vi "Dashboard Main.vi"() -> ()   [LabVIEW 2015]
uses:
  Vision/Vision Support Code/Camera Types.ctl
  <vilib>/Rock Robotics/WPI/Camera/WPI_CameraImageSize.ctl
  <vilib>/Utility/miscctls.llb/LVRowAndColumnTypeDef.ctl
  <vilib>/event_ctls.llb/eventvkey.ctl
  <vilib>/Rock Robotics/WPI/Dashboard/WPI_DashboardLogging Global.vi
  Vision/Robot Global Data.vi
  <vilib>/Rock Robotics/Network Tables/NT Read Numeric Array.vi
  <vilib>/Rock Robotics/Network Tables/NT Read Boolean.vi
  <vilib>/Rock Robotics/Network Tables/NT Write Boolean.vi
  <vilib>/Utility/config.llb/Write Key (String).vi
  <vilib>/Utility/config.llb/Write Key (I32).vi
  <vilib>/Utility/config.llb/NI_LVConfig.lvlib
  <vilib>/vision/NI_Vision_Development_Module.lvlib
panel:
  in  "Tab Control":T1(tab)
  out "Boolean 4":bool
  out "Boolean 3":bool
  out "Boolean 2":bool
  out "Boolean":bool
  out "Original Image":T2(plugin-control)
  out "Masked":T2(plugin-control)
  out "Detected Targets":T3(array[cluster]) {"Normalized Rect"."Numeric 5" format="%#_2g"; "Normalized Rect"."Numeric 3" format="%#_2g"; "Normalized Rect"."Numeric 2" format="%#_2g"; "Normalized Rect"."Numeric" format="%#_2g"}
  out "Sorted Particle Scores":T4(array[cluster]) {"Moment Factor" format="%#_3g"; "Aspect Ratio" format="%#_3g"; "Area to CH" format="%#_3g"; "X" format="%#_3g"; "Y" format="%#_3g"}
  in  "LED Color":T5={"Hue"={98.0, 128.0}, "Sat"={64.0, 255.0}, "Val"={48.571428571428584, 255.0}} {"Hue" scale=0.0..255.0 scale format="%#_3g"}
  in  "Display Original":bool=TRUE
  in  "Display Mask":bool=TRUE
  in  "Emphasize Limit Tests":bool=TRUE
  in  "Camera Type":T6=enum."MS HD3000 square"
  in  "Aspect Fudge Factor":dbl=1.0
  in  "Score Threshold":dbl=75.0
  in  "Image Size":T7=enum."320x240"
  out "Qualified Particles":i32
  out "Highest Avg Score":dbl
  in  "Min Score Threshold":i32=75
  out "NT Connection":bool
  out "fps":dbl format="%#.1g"
  out "Mbps":dbl format="%#.1g"
  out "Mbps LED":bool
  in  "TCP":refnum<k5>
  in  "Rec Mode":enum32{"Stop", "Record", "Playback"}(radio)
  in  "Vision":u16(ring)=2 items=["Camera Off", "USB Camera SW", "USB Camera HW", "IP Camera"]
  out "Camera IP":string
  out "Image Message":string="Timeout in Camera Communications"
  in  "Dashboard Tab":T8(tab)
  out "Ball Holder OR":bool
  out "Shooter":bool
  out "Intake":bool
  in  "Gyro Reset":bool
  out "Gyro":dbl
  in  "OW Arm Angle":dbl=42.0
  out "Wheels Good":bool
  out "Arm Good":bool
  in  "Auto Selection":u16(ring) caption="Menu Ring" items=["Do Nothing", "Bump", "CDF", "Low Bar", "Bump - SHOOT", "Bump - SHOOT DRIVE", "CDF - SHOOT", "Low Bar - SHOOT", "Spy - SHOOT", "Misc Auto 1"]
  out "VISION GOOD":bool
  out "Arm Angle":dbl
  out "Encoder Distance":dbl
  out "RPM L":dbl
  out "RPM R":dbl
  out "RPM SP":dbl
  out "Angle SP":dbl
  out "Found Targets":cluster{dbl, dbl}
  in  "Vision Good Range":dbl=0.05
  in  "Vision Scaling":dbl
  in  "148 Arm Angle":dbl=60.0
  out "Encoder Gyro":dbl
  out "Gyro":dbl(knob) scale=0.0..360.0
  in  "D4 Wheel Speed":dbl=5000.0
  in  "Fender Wheel Speed":dbl=4999.0
  in  "Select Auto":string(combo)
  in  "Camera Settings":T9={"Frame Rate"=30, "Compression"=30, "Size"=1} {"Frame Rate" scale=1.0..30.0; "Size" items=["640x480", "320x240", "160x120"]}
  out "MotorChart R":cluster{"Numeric":dbl, "Numeric":dbl}(graph)
  out "MotorChart L":T10(graph)
  out "MotorSliders R":cluster{"MotorSlide1":dbl, "MotorSlide2":dbl} {"MotorSlide2" scale=-1.0..1.0 scale format="%#_2e"; "MotorSlide1" scale=-1.0..1.0 scale format="%#_2e"}
  out "MotorSliders L":T11 {"MotorSlide4 2" scale=0.0..14.0 scale format="%#_2e"; "MotorSlide2" scale=-1.0..1.0 scale format="%#_2e"; "MotorSlide1" scale=-1.0..1.0 scale format="%#_2e"}
  out "JS1 Z":dbl(slide) scale=-1.0..1.0 scale format="%#_2e"
  out "JS1 Graph":cluster{"X":dbl, "Y":dbl}[](graph)
  out "JS1 Buttons":T12
  out "JS2 Z":dbl(slide) scale=-1.0..1.0 scale format="%#_2e"
  out "JS2 Graph":cluster{"X":dbl, "Y":dbl}[](graph)
  out "JS2 Buttons":T12
  out "Mode":T13(ring)=enum."Auto Disabled"
  in  "DB Camera Config":bool
  in  "DB/String 9":string
  in  "DB/String 8":string
  in  "DB/String 7":string
  in  "DB/String 6":string
  in  "DB/String 5":string
  in  "DB/String 4":string
  in  "DB/String 3":string
  in  "DB/String 2":string
  in  "DB/String 1":string
  in  "DB/String 0":string
  in  "DB/Slider 0":dbl(slide) scale=0.0..5.0
  in  "DB/Slider 1":dbl(slide) scale=0.0..5.0
  in  "DB/Slider 2":dbl(slide) scale=0.0..5.0
  in  "DB/Slider 3":dbl(slide) scale=0.0..5.0
  out "DB/LED 3":bool
  out "DB/LED 2":bool
  out "DB/LED 1":bool
  out "DB/LED 0":bool
  in  "DB/Button 3":bool
  in  "DB/Button 2":bool
  in  "DB/Button 1":bool
  in  "DB/Button 0":bool caption="New Name"
  in  "Test Slider":dbl(slide) scale=0.0..100.0 scale format="%#_3g"
  in  "On/Off":bool caption="Solenoid"
  in  "Test Name":u16(ring) items=["Select the test to run..."]
  in  "Test Tree":string(tree)
  in  "Motor":cluster{"Value":dbl, "Enable":bool} {"Value" scale=-1.0..1.0 scale format="%#_3g"}
  out "Progress":T14 {"Test Progress" scale=0.0..100.0}
  in  "Rev/Fwd":cluster{"Forward":bool, "Reverse":bool}
  in  "Test Ring":u16(ring) items=["Monochrome", "Color"]
  out "Cmd Status":string
  in  "Execute Command":bool
  in  "Command Params":string[][](table)
  in  "Command Selection":i32(listbox)
  in  "CheckList":i32(listbox)
  out "Tree":string(tree)
  # "Density Profile"
  # "Left"
  # "Front"
  # "Right"
  # "Battery"
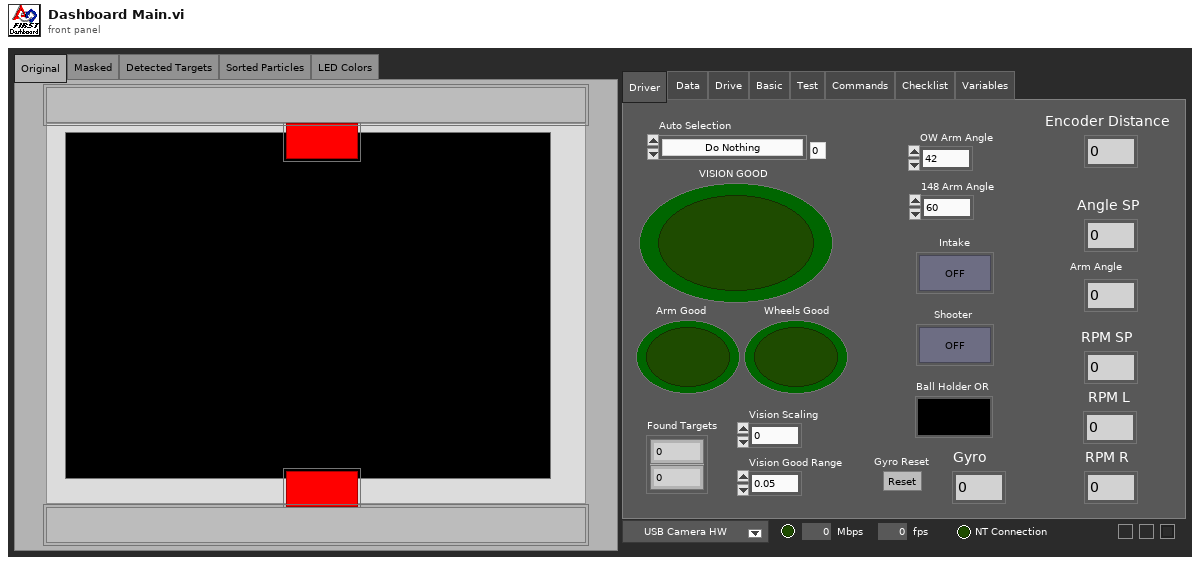
[diagram p1: front panel]
types:
  T1 = enum32{"Original", "Masked", "Detected Targets", "Sorted Particles", "LED Colors"}
  T2 = typedef "IMAQ Image.ctl" = refnum<image>
  T3 = cluster{"Distance (ft)":dbl, "Center":cluster{dbl, dbl}, "Normalized Rect":cluster{"Numeric":dbl, "Numeric 2":dbl, "Numeric 3":dbl, "Numeric 5":dbl}}[]
  T4 = cluster{"Rectangle px":cluster{"Numeric":dbl, "Numeric 2":dbl, "Numeric 3":dbl, "Numeric 5":dbl}, "Aspect Ratio":dbl, "Area to CH":dbl, "X":dbl, "Y":dbl, "Moment Factor":dbl}[]
  T5 = cluster{"Hue":cluster{dbl, dbl}, "Sat":cluster{dbl, dbl}, "Val":cluster{dbl, dbl}}
  T6 = typedef "Camera Types.ctl" = enum16{"206", "1011", "1013", "MS HD3000 square", "MS HD3000 640x480"}
  T7 = typedef "WPI_CameraImageSize.ctl" = enum16{"640x480", "320x240", "160x120", "Custom"}
  T8 = enum32{"Driver", "Data ", "Drive", "Basic", "Test", "Commands", "Checklist", "Variables"}
  T9 = cluster{"Frame Rate":i32, "Compression":i32, "Size":u16}
  T10 = cluster{"Numeric":dbl, "Numeric":dbl, "Battery V":dbl}
  T11 = cluster{"MotorSlide1":dbl, "MotorSlide2":dbl, "MotorSlide4 2":dbl}
  T12 = cluster{bool, bool, bool, bool, bool, bool, bool, bool, bool, bool, bool, bool}
  T13 = enum8{"Tele-Op Disabled", "Tele-Op Enabled", "Auto Disabled", "Auto Enabled", "Test Disabled", "Test Enabled", "Disconnected", "No Code", "E-Stop"}
  T14 = cluster{"Test Progress":u8, "Test Progress Text":string}
  T15 = typedef "Image Type" = u32
  T16 = typedef "Particle Parameters" = i32
  T17 = cluster{"IDs":cluster{"RPC field ID":u16, "Unique ID":u16}, "String":string}
  T18 = enum32{"Drive", "Basic", "Custom", "Test", "Checklist", "Variables"}
  T19 = cluster{"Bounding box":cluster{"left":dbl, "top":dbl, "right":dbl, "bottom":dbl}, "Aspect Ratio":dbl, "Area to CH":dbl, "X Mask":dbl, "Y Mask":dbl, "Moment":dbl}[]
  T20 = cluster{"Rectangle":cluster{"Numeric":dbl, "Numeric 2":dbl, "Numeric 3":dbl, "Numeric 5":dbl}, "L":dbl, "Area to CH":dbl, "X":dbl, "Y":dbl, "Moment Factor":dbl}[]
  T21 = cluster{"Found Targets[0]":cluster{"Distance (ft)":dbl, "Center":cluster{dbl, dbl}, "Normalized Rect":cluster{"Numeric":dbl, "Numeric 2":dbl, "Numeric 3":dbl, "Numeric 5":dbl}}, "Found Targets[1]":cluster{"Distance (ft)":dbl, "Center":cluster{dbl, dbl}, "Normalized Rect":cluster{"Numeric":dbl, "Numeric 2":dbl, "Numeric 3":dbl, "Numeric 5":dbl}}, "Found Targets[2]":cluster{"Distance (ft)":dbl, "Center":cluster{dbl, dbl}, "Normalized Rect":cluster{"Numeric":dbl, "Numeric 2":dbl, "Numeric 3":dbl, "Numeric 5":dbl}}, "Found Targets[3]":cluster{"Distance (ft)":dbl, "Center":cluster{dbl, dbl}, "Normalized Rect":cluster{"Numeric":dbl, "Numeric 2":dbl, "Numeric 3":dbl, "Numeric 5":dbl}}, "Found Targets[4]":cluster{"Distance (ft)":dbl, "Center":cluster{dbl, dbl}, "Normalized Rect":cluster{"Numeric":dbl, "Numeric 2":dbl, "Numeric 3":dbl, "Numeric 5":dbl}}, "Found Targets[5]":cluster{"Distance (ft)":dbl, "Center":cluster{dbl, dbl}, "Normalized Rect":cluster{"Numeric":dbl, "Numeric 2":dbl, "Numeric 3":dbl, "Numeric 5":dbl}}, "Found Targets[6]":cluster{"Distance (ft)":dbl, "Center":cluster{dbl, dbl}, "Normalized Rect":cluster{"Numeric":dbl, "Numeric 2":dbl, "Numeric 3":dbl, "Numeric 5":dbl}}, "Found Targets[7]":cluster{"Distance (ft)":dbl, "Center":cluster{dbl, dbl}, "Normalized Rect":cluster{"Numeric":dbl, "Numeric 2":dbl, "Numeric 3":dbl, "Numeric 5":dbl}}, "Found Targets[8]":cluster{"Distance (ft)":dbl, "Center":cluster{dbl, dbl}, "Normalized Rect":cluster{"Numeric":dbl, "Numeric 2":dbl, "Numeric 3":dbl, "Numeric 5":dbl}}}
  T22 = typedef "NI_LVConfig.lvlib/Config Data RefNum.ctl" = refnum<k1>
  T23 = cluster{"Error Strings":string, "Disable Counts":cluster{u16, u16}, "Rail Faults":cluster{u16, u16, u16}, "Robot IP":string, "DB Mode":u8, "Event Info":cluster{"Name":string, "Type":u8, "Number":u16, "Replay":u8}, "Camera Addr":string}
  T24 = cluster{"Storage":cluster{"Disk Free":u64, "RAM Block":u32, "RAM free":u32}, "CPU Utilization":cluster{"CPU % ISR":sgl, "CPU % Time Crit":sgl, "CPU % Timed Str":sgl, "CPU % High":sgl, "CPU % Above":sgl, "CPU % Normal":sgl, "CPU % Low":sgl}, "CAN":cluster{"% Bus Utilization":sgl, "Bus Off Cnt":u32, "TX_FIFO Full Cnt":u32, "Receive Error Cnt":u8, "Transmit Error Cnt":u8}, "HID":cluster{"HID Outputs":u32, "Rumble Low":u16, "Rumble High":u16}[]}
  T25 = cluster{"Status bits":cluster{"Test Mode":bool, "Autonomous":bool, "Enabled":bool, "Code Start":bool, "Brownout":bool, "Reserved 2":bool, "Reserved 3":bool, "E-Stop":bool}, "Code Trace":cluster{"Disabled":bool, "TeleOp":bool, "Auto":bool, "Test":bool}, "Controller Type":enum16{"unknown", "cRIO", "roboRio"}, "Code?":enum16{"unknown", "noCode", "code"}, "Battery V":dbl}
  T26 = cluster{"Control Bits":cluster{"TestMode":bool, "Autonomous":bool, "Enabled":bool, "FMS Present":bool, bool, bool, bool, "E-Stop":bool}, "Team Station ":u8, "Countdown":sgl, "Joystick Values":cluster{"Axes":dbl[], "Buttons":bool[], "POVs":i16[]}[]}
  T27 = cluster{"Axes":dbl[], "Buttons":bool[], "POVs":i16[]}[]
  T28 = cluster{"Axes":dbl[], "Buttons":bool[], "POVs":i16[]}
  T29 = cluster{"Buttons[0]":bool, "Buttons[1]":bool, "Buttons[2]":bool, "Buttons[3]":bool, "Buttons[4]":bool, "Buttons[5]":bool, "Buttons[6]":bool, "Buttons[7]":bool, "Buttons[8]":bool, "Buttons[9]":bool, "Buttons[10]":bool, "Buttons[11]":bool}
  T30 = cluster{"Operation":enum16{"Update", "Clear"}, "Color Box":u32}[]
  T31 = typedef "eventvkey.ctl" = enum16{"ASCII", "Enter", "Return", "Shift", "Ctrl", "Alt", "Cmd", "Opt", "Caps", "NumLock", "Clear", "Break", "Up", "Down", "Left", "Right", "Insert", "Delete", "Home", "End", "PageUp", "PageDown", "Escape", "Help", "Pause", "ScrollLock", "F1", "F2", "F3", "F4", "F5", "F6", "F7", "F8", "F9", "F10", "F11", "F12", "F13", "F14", "F15", "F16", "F17", "F18", "F19", "F20", "F21", "F22", "F23", "F24", "Play", "VolumeUp", "VolumeDown", "Mute", "Two Byte Char"}
  T32 = cluster{"Image Size":bool, "Image Type":bool, "Pixel Value":bool, "ROI Information":bool, "Zoom Factor":bool}
  T33 = enum8{"Enabled", "Disabled", "Disabled and Grayed Out"}
  T34 = cluster{"Operation":enum16{"Update", "Clear"}, "Color Box":u32}
  T35 = typedef "LVRowAndColumnTypeDef.ctl" = cluster{"Row":i32, "Column":i32}
  T36 = cluster{"Shift":bool, "Ctrl":bool, "Alt":bool, "Cmd":bool, "Opt":bool}
  T37 = enum32{"Drive", "Basic", "Custom", "Test", "Commands", "Checklist", "Variables"}
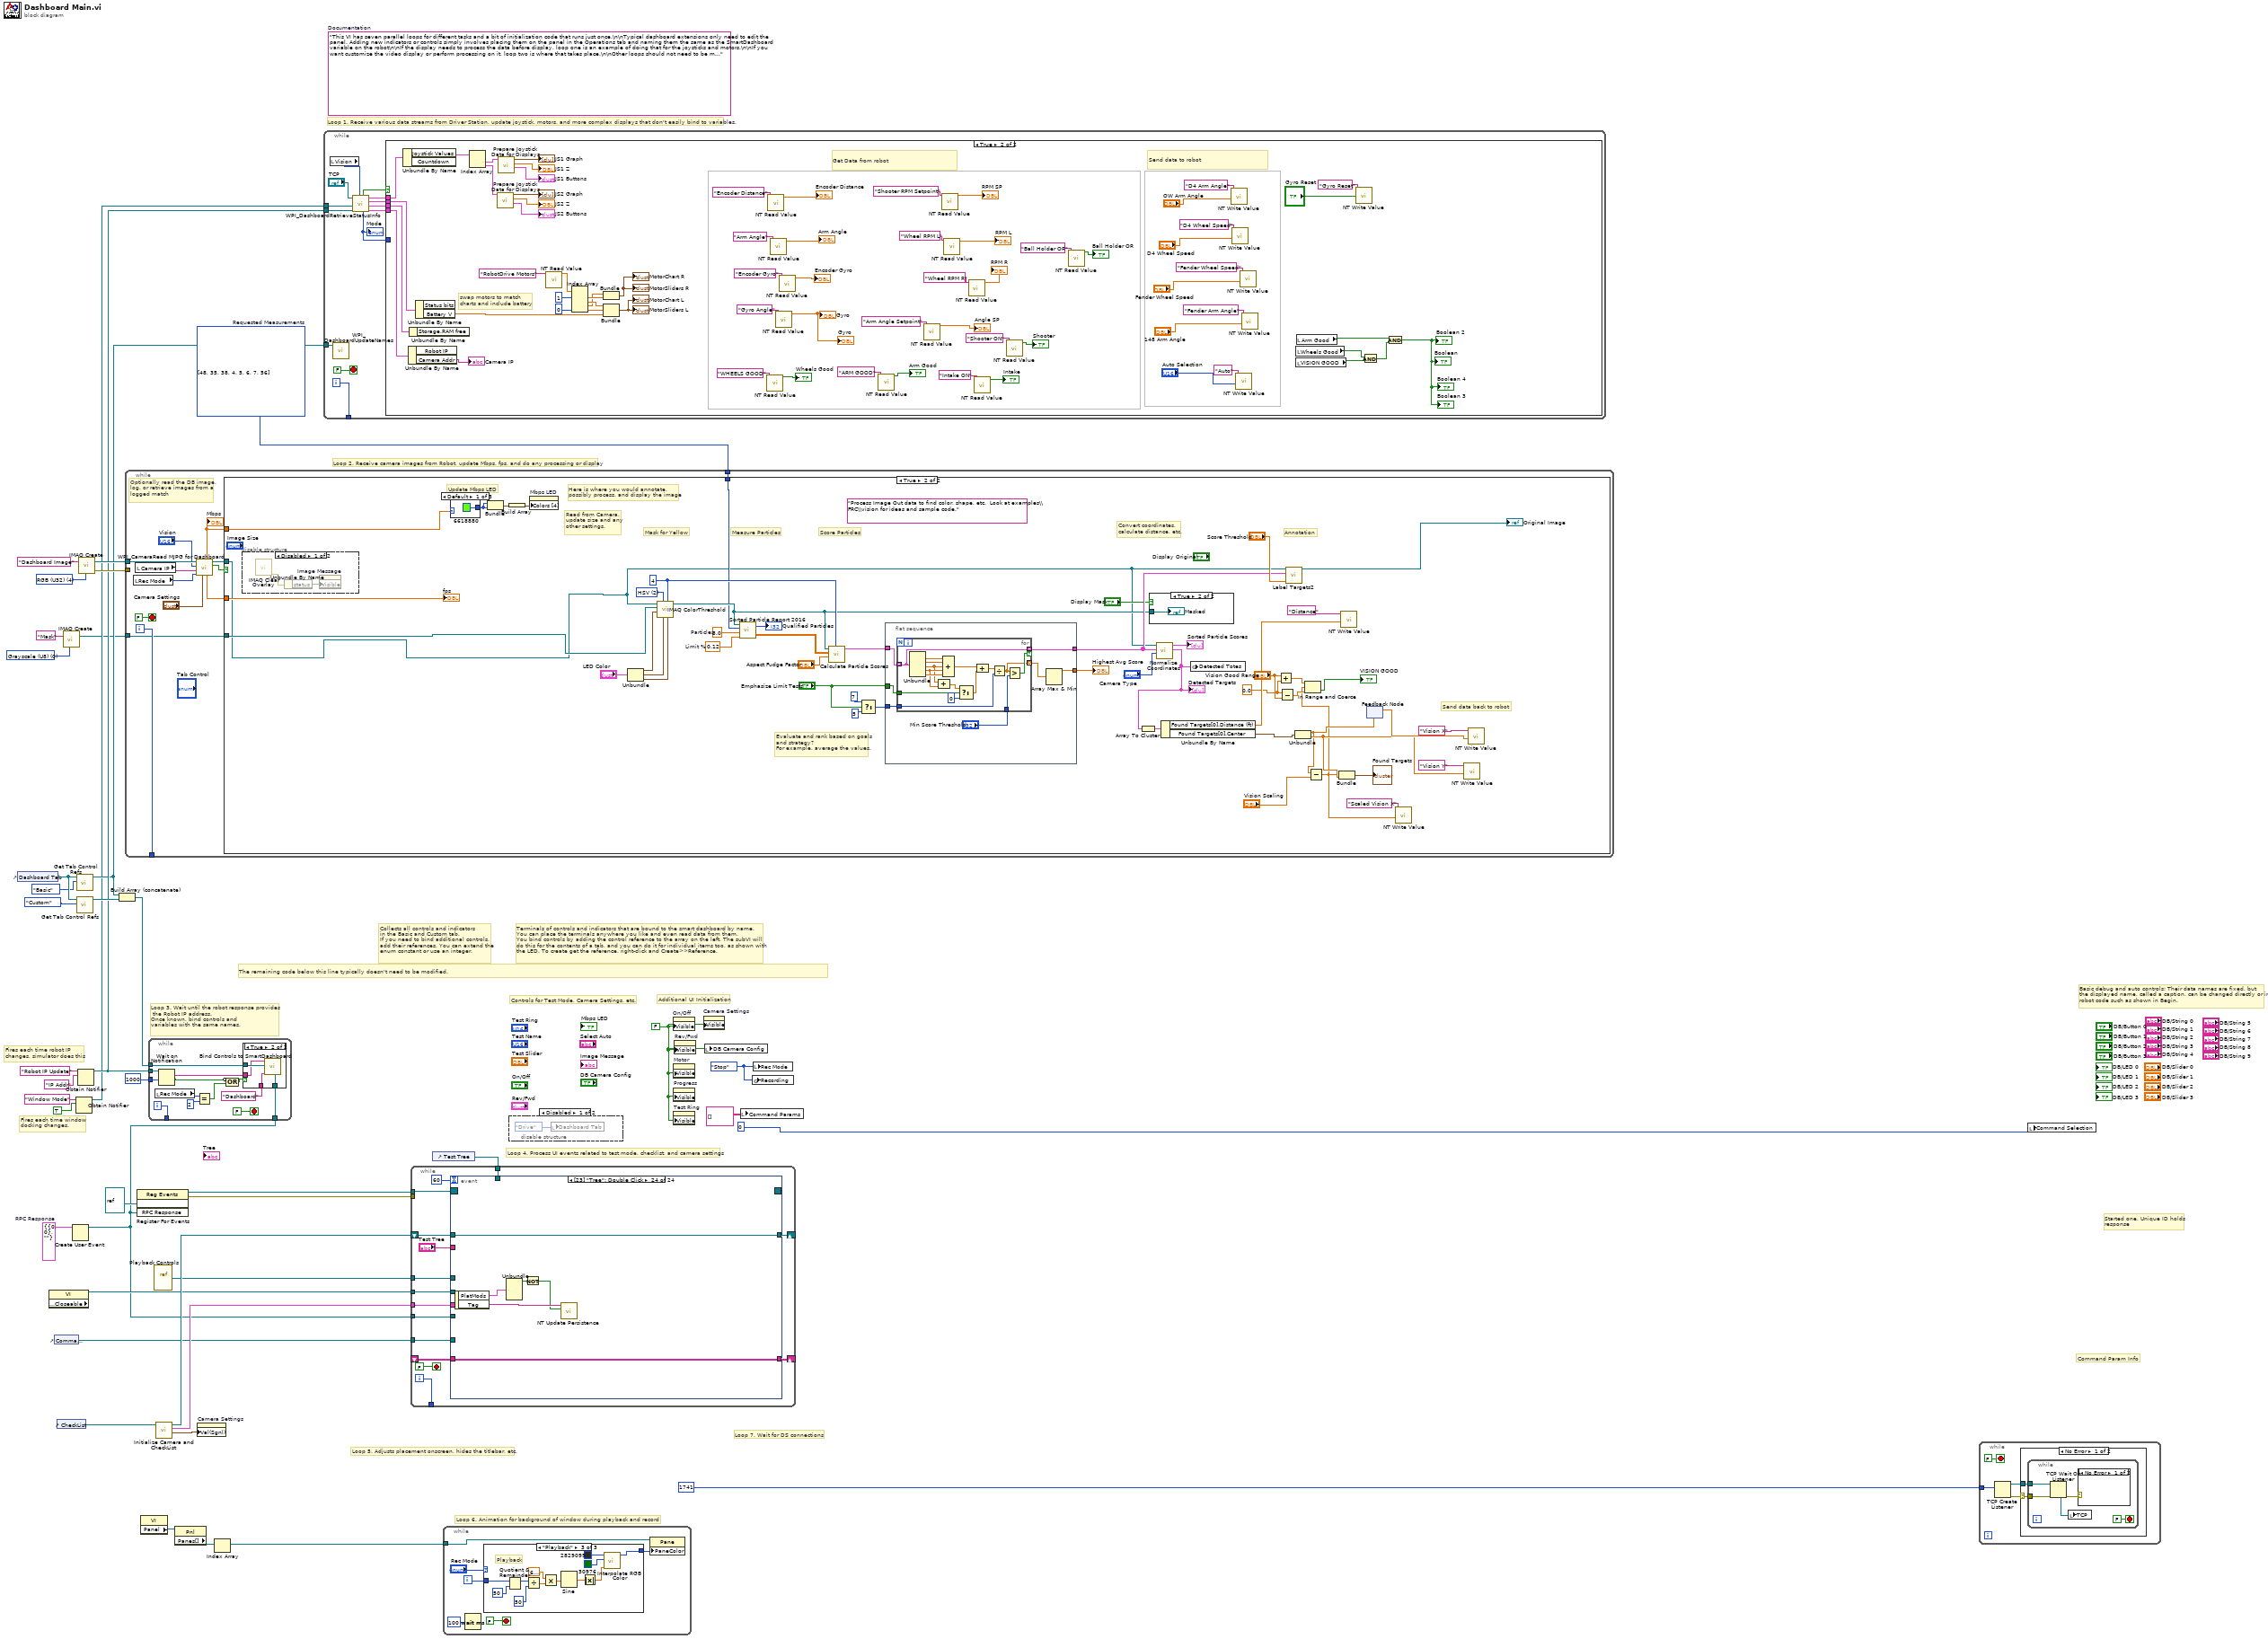
[diagram p0: block diagram]
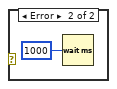
[diagram p3: hidden frame]
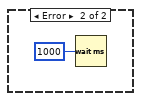
[diagram p4: hidden frame]
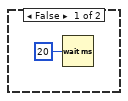
[diagram p5: hidden frame]
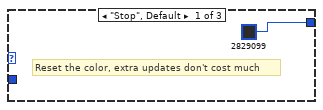
[diagram p6: hidden frame]
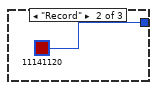
[diagram p7: hidden frame]
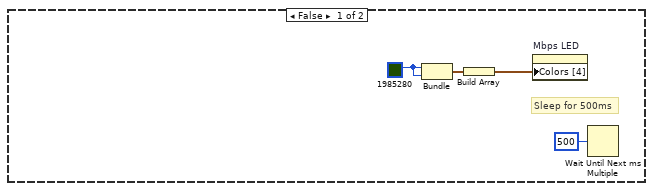
[diagram p9: hidden frame]
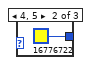
[diagram p12: hidden frame]
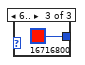
[diagram p13: hidden frame]
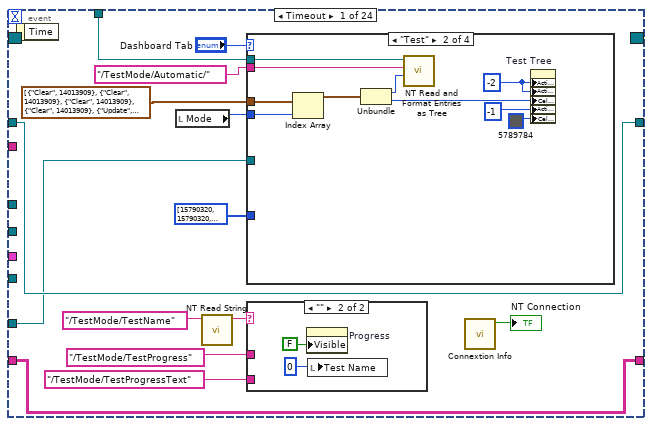
[diagram p14: hidden frame]
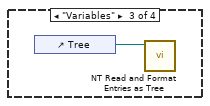
[diagram p16: hidden frame]
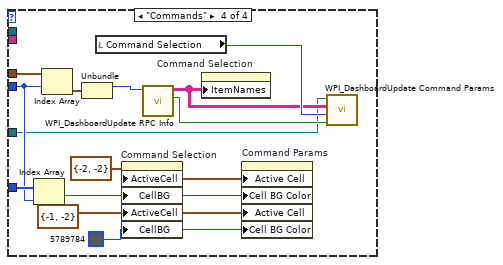
[diagram p17: hidden frame]
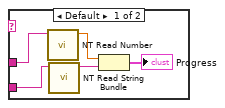
[diagram p18: hidden frame]
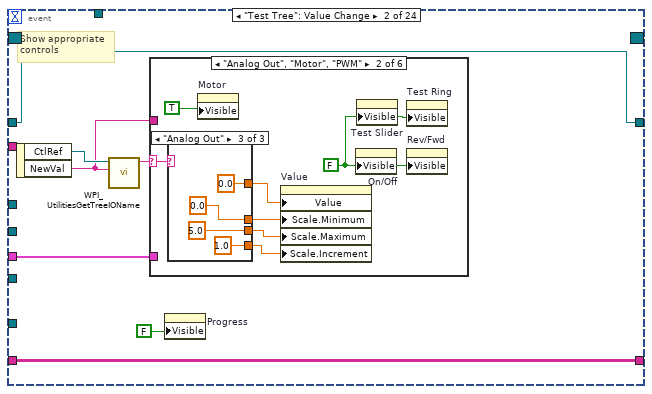
[diagram p19: hidden frame]
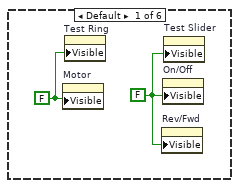
[diagram p20: hidden frame]
diagram:
  w3 = T15 0 items=["Grayscale (U8)", "Grayscale (I16)", "Grayscale (SGL)", "Complex (CSG)", "RGB (U32)", "HSL (U32)", "RGB (U64)", "Grayscale (U16)"] ("Image Type")
  w1 = T16[] [48, 35, 38, 4, 5, 6, 7, 56] items=["Center of Mass X", "Center of Mass Y", "First Pixel X", "First Pixel Y", "Bounding Rect Left", "Bounding Rect Top", "Bounding Rect Right", "Bounding Rect Bottom", "Max Feret Diameter Start X", "Max Feret Diameter Start Y", "Max Feret Diameter End X", "Max Feret Diameter End Y", "Max Horiz. Segment Length Left", "Max Horiz. Segment Length Right", "Max Horiz. Segment Length Row", "-", "Bounding Rect Width", "Bounding Rect Height", "Bounding Rect Diagonal", "Perimeter", "Convex Hull Perimeter", "Holes' Perimeter", "Max Feret Diameter", "Equivalent Ellipse Major Axis", "Equivalent Ellipse Minor Axis", "Equivalent Ellipse Minor Axis (Feret)", "Equivalent Rect Long Side", "Equivalent Rect Short Side", "Equivalent Rect Diagonal", "Equivalent Rect Short Side (Feret)", "Average Horiz. Segment Length", "Average Vert. Segment Length", "Hydraulic Radius", "Waddel Disk Diameter", "-", "Area", "Holes' Area", "Particle & Holes' Area", "Convex Hull Area", "Image Area", "-", "Number of Holes", "Number of Horiz. Segments", "Number of Vert. Segments", "-", "Orientation", "Max Feret Diameter Orientation", "-", "% Area/Image Area", "% Area/(Particle & Holes' Area)", "Ratio of Equivalent Ellipse Axes", "Ratio of Equivalent Rect Sides", "-", "Elongation Factor", "Compactness Factor", "Heywood Circularity Factor", "Type Factor", "-", "Sum X", "Sum Y", "Sum XX", "Sum XY", "Sum YY", "Sum XXX", "Sum XXY", "Sum XYY", "Sum YYY", "-", "Moment of Inertia XX", "Moment of Inertia XY", "Moment of Inertia YY", "Moment of Inertia XXX", "Moment of Inertia XXY", "Moment of Inertia XYY", "Moment of Inertia YYY", "Norm. Moment of Inertia XX", "Norm. Moment of Inertia XY", "Norm. Moment of Inertia YY", "Norm. Moment of Inertia XXX", "Norm. Moment of Inertia XXY", "Norm. Moment of Inertia XYY", "Norm. Moment of Inertia YYY", "Hu Moment 1", "Hu Moment 2", "Hu Moment 3", "Hu Moment 4", "Hu Moment 5", "Hu Moment 6", "Hu Moment 7"]  # Requested Measurements
  w9 = T17 {"IDs"={"RPC field ID"=0, "Unique ID"=0}, "String"=""}  # RPC Response
  w22 = enum32{"Stop", "Record", "Playback"}."Stop" ("Rec Mode")
  w14 = FALSE ("Visible")
  (unwired) "This VI has seven parallel loops for different tasks and a bit of initialization code that runs just once.\n\nTypical dashboard extensions only need to edit the panel. Adding new indicators or controls simply involves placing them on the panel in the Operations tab and naming them the same as the SmartDashboard variable on the robot\n\nIf the display needs to process the data before display, loop one is an example of doing that for the joysticks and motors.\n\nIf you want customize the video display or perform processing on it, loop two is where that takes place.\n\nOther loops should not need to be modified. They are pretty standard, and document the task they perform."  # Documentation
  w42 = T15 4 items=["Grayscale (U8)", "Grayscale (I16)", "Grayscale (SGL)", "Complex (CSG)", "RGB (U32)", "HSL (U32)", "RGB (U64)"] ("Image Type")
  # "Command Param Info"
  # "Started one, Unique ID holds\nresponse"
  # "Loop 7. Wait for DS connections"
  # "Basic debug and auto controls: Their data names are fixed, but\nthe displayed name, called a caption, can be changed directly or in\nrobot code such as shown in Begin."
  # "Controls for Test Mode, Camera Settings, etc."
  # "Additional UI Initialization"
  # "Loop 6. Animation for background of window during playback and record"
  # "Fires each time robot IP\nchanges, simulator does this"
  # "Fires each time window\ndocking changes."
  # "Collects all controls and indicators\nin the Basic and Custom tab.\nIf you need to bind additional controls,\nadd their references. You can extend the\nenum constant or use an integer."
  # "The remaining code below this line typically doesn't need to be modified."
  # "Loop 4. Process UI events related to test mode, checklist, and camera settings"
  # "Terminals of controls and indicators that are bound to the smart dashboard by name.\nYou can place the terminals anywhere you like and even read data from them.\nYou bind controls by adding the control reference to the array on the left. The subVI will\ndo this for the contents of a tab, and you can do it for individual items too, as shown with\nthe LED. To create get the reference, right-click and Create>>Reference."
  # "Loop 3. Wait until the robot response provides\n the Robot IP address.\nOnce known, bind controls and\nvariables with the same names."
  # "Loop 5. Adjusts placement onscreen, hides the titlebar, etc."
  # "Loop 1. Receive various data streams from Driver Station, update joystick, motors, and more complex displays that don't easily bind to variables."
  # "Loop 2. Receive camera images from Robot, update Mbps, fps, and do any processing or display"
  n1 = control-ref of="Dashboard Tab"() -> (w20:refnum<vi>)
  n2 = property class="VI" props=["Front Panel.Closeable"]() -> (reference out=w21:refnum<vi>)  [unwired: 2 in, 2 out]
  n3 = control-ref of="Command Params"() -> (w5:refnum<vi>)
  n4 = control-ref of="CheckList"() -> (w15:refnum<vi>)
  n5 = call "IMAQ Create"("Image Name"="Mask", "Image Type"=w3) -> ("New Image"=w2:T2)  [unwired: 2 in, 2 out]
  n6 = Create User Event(user event datatype=w9) -> (user event=w6:refnum<user-event>)  [unwired: 1 in, 1 out]
  n7 = Obtain Notifier(name (unnamed)="Window Mode", notification data type=TRUE) -> (notifier out=w11:refnum<notifier>)  [unwired: 2 in, 2 out]
  n8 = call <vilib>:"Get Tab Control Refs.vi"("Page Index"=T18."Basic" ("Dashboard Tab"), "TabControl in"=w20) -> ("ControlsOnPage"=w12:refnum<vi>[])  [unwired: 9 in]
  n9 = call <vilib>:"Get Tab Control Refs.vi"("Page Index"=T18."Custom" ("Dashboard Tab"), "TabControl in"=w20) -> ("ControlsOnPage"=w19:refnum<vi>[])  [unwired: 9 in]
  n10 = Obtain Notifier(name (unnamed)="Robot IP Update", notification data type="IP Addr" ("name (unnamed)")) -> (notifier out=w13:refnum<notifier>)  [unwired: 2 in, 2 out]
  n11 = call "IMAQ Create"("Image Name"="Dashboard Image", "Image Type"=w42) -> ("New Image"=w40:T2, "error out"=w39:errorcluster)  [unwired: 2 in, 1 out]
  n12 = Build Array (concatenate)(w12, w19) -> (w18:refnum<vi>[])
  n13 = while {
    tunnel: w40 -> [w53]
    tunnel: w39 -> [_]
    tunnel: [w54] -> _
    tunnel: w2 -> [w44]
    tunnel: w1 -> [w43]
    i -> [w54]
    stop <- FALSE stop-if-true
    # "Optionally read the DB image,\nlog, or retrieve images from a\nlogged match"
    n14 = local read "Rec Mode"() -> (w48:enum32{"Stop", "Record", "Playback"})
    n15 = local read "Camera IP"() -> (w46:string)
    n16 = call <vilib>:"WPI_CameraRead MJPG for Dashboard.vi"("Camera Settings"="Camera Settings", "Rec Mode"=w48, "Camera IP"=w46, "Camera Mode"="Vision", "Refnum in"=w53) -> ("Active"=w51:bool, "Refnum out"=w52:T2, "FPS"=w50:dbl, "Bandwidth (Mbps)"=w45:dbl)  [unwired: 3 in]
    "Mbps" <- w45
    n17 = case shown="True" w51 {
      tunnel: w52 -> [_ w60]
      tunnel: w45 -> [_ w107]
      tunnel: w50 -> [_ w106]
      tunnel: w44 -> [_ w68]
      tunnel: w43 -> [_ w82]
      frame False {
        w56 = u32 1985280 ("Color Box")
        # "Sleep for 500ms"
        n18 = Bundle("Color Box"=w56, "Color Box"=w56) -> (w58:cluster{"Color Box":u32, "Color Box":u32})  [unwired: 1 out]
        n19 = Build Array(w58) -> (w57:cluster{"Color Box":u32, "Color Box":u32}[])
        n20 = property on="Mbps LED" class="Bool (strict)"("Colors [4]"=w57) -> ()  [unwired: 2 in, 2 out]
        n21 = Wait Until Next ms Multiple(millisecond multiple=u32 500) -> ()  [unwired: 1 out]
      }
      frame True {
        w73 = 0.0 ("x")
        w104 = 4 ("Replace Value")
        w91 = u16 2 items=["RGB", "HSL", "HSV", "HSI"] ("Color Mode")
        (unwired) "Process Image Out data to find color, shape, etc.  Look at examples\\FRC\\vision for ideas and sample code."
        w89 = 0.12  # Limit %
        w87 = 3.0  # Particles
        # "Send data back to robot"
        # "Evaluate and rank based on goals\nand strategy?\nFor example, average the values."
        # "Read from Camera,\nupdate size and any\nother settings."
        # "Measure Particles"
        # "Convert coordinates,\ncalculate distance, etc."
        # "Annotation"
        # "Score Particles"
        # "Mask for Yellow"
        # "Here is where you would annotate,\npossibly process, and display the image"
        # "Update Mbps LED"
        n22 = disable-structure shown="Disabled" {
          frame Disabled {
            n23 = call "IMAQ Clear Overlay"() -> ("error out"=w111:errorcluster)  [unwired: 3 in, 8 out]
            n24 = Unbundle By Name(w111) -> ("status"=w112:bool)
            n25 = property on="Image Message" class="Str"("Visible"=w112) -> ()  [unwired: 2 in, 2 out]
          }
          frame Enabled {
          }
        }
        n26 = case shown="Default" w107 {
          tunnel: [u32 6618880 ("Color Box") u32 16776722 ("Color Box") u32 16716800 ("Color Box")] -> w108
          frame Default {
          }
          frame 4, 5 {
          }
          frame 6.. {
          }
        }
        n27 = Bundle("Color Box"=w108, "Color Box"=w108) -> (w110:cluster{"Color Box":u32, "Color Box":u32})  [unwired: 1 out]
        n28 = Build Array(w110) -> (w109:cluster{"Color Box":u32, "Color Box":u32}[])
        n29 = property on="Mbps LED" class="Bool (strict)"("Colors [4]"=w109) -> ()  [unwired: 2 in, 2 out]
        n30 = Unbundle("LED Color") -> ("Hue"=w83:cluster{dbl, dbl}, "Sat"=w84:cluster{dbl, dbl}, "Val"=w85:cluster{dbl, dbl})
        n31 = call "IMAQ ColorThreshold"("Blue or Luma or Val or Inten Range"=w85, "Replace Value"=w104, "Green or Sat Range"=w84, "Color Mode"=w91, "Red or Hue Range"=w83, "Image Dst"=w68, "Image Src"=w60) -> ("Image Dst Out"=w92:T2)  [unwired: 3 in, 1 out]
        n32 = call "Sorted Particle Report 2016.vi"("Min Area Size %"=w89, "Particle Count Limit"=w87, "Pixel Measurements"=w82, "Image in"=w92) -> ("Sorted Data"=w93:dbl[][], "Particles"=→"Qualified Particles":i32)
        n33 = call "Calculate Particle Scores.vi"("Pixel Value"=w104, "Aspect Fudge Factor"="Aspect Fudge Factor", "Sorted Data"=w93, "Image in"=w92) -> ("Scores"=w95:T19)  [unwired: 7 in]
        n34 = Select(t=7, s="Emphasize Limit Tests", f=5) -> (s? t:f=w98:i32)
        n35 = flat-sequence {
          tunnel: w95 -> [w119]
          tunnel: w98 -> [w117]
          tunnel: [w120] -> w99
          tunnel: [w114] -> w102
          tunnel: "Emphasize Limit Tests" -> [w118]
          frame #0 {
            n36 = for {
              tunnel: w119 -> [w134] mode=indexing
              tunnel: [w134] -> w114 mode=indexing if=w133
              tunnel: [w132] -> w115 mode=indexing
              tunnel: w117 -> [w131]
              tunnel: "Min Score Threshold" -> [w130]
              tunnel: w118 -> [w123]
              n37 = Unbundle(w134) -> ("Aspect Ratio"=w136:dbl, "Area to CH"=w135:dbl, "X Mask"=w125:dbl, "Y Mask"=w126:dbl, "Moment"=w127:dbl)  [unwired: 1 out]
              n38 = Compound Arithmetic op=ADD(w125, w126) -> (w124:dbl)
              n39 = Compound Arithmetic op=ADD(w136, w135, w125, w126, w127) -> (w129:dbl)
              n40 = Select(t=w124, s=w123, f=0) -> (s? t:f=w122:dbl)
              n41 = Compound Arithmetic op=ADD(w129, w122) -> (w128:dbl)
              n42 = Divide(x=w128, y=w131) -> (x/y=w132:dbl)
              n43 = Greater?(x=w132, y=w130) -> (0:w133:bool)
            }
            n44 = Array Max & Min(array=w115) -> (max value=w120:dbl)  [unwired: 3 out]
          }
        }
        n45 = case shown="True" "Display Mask" {
          tunnel: w92 -> [_ w113]
          frame False {
          }
          frame True {
            "Masked" <- w113
          }
        }
        n46 = call "Normalize Coordinates.vi"("Camera Type"="Camera Type", "Targets"=w102, "Image in"=w60) -> ("Found Targets"=w80:T3, "Sorted Scores"=→"Sorted Particle Scores":T20)  [unwired: 7 in]
        "Detected Targets" <- w80
        n47 = Array To Cluster(array=w80) -> (cluster=w81:T21)
        n48 = Unbundle By Name(w81) -> ("Found Targets[0].Distance (ft)"=w78:dbl, "Found Targets[0].Center"=w79:cluster{dbl, dbl})
        n49 = global write "Robot Global Data.vi" "Detected Totes"(w80) -> ()
        n50 = Add(x="Vision Good Range", y=w73) -> (x+y=w71:dbl)
        n51 = Subtract(x=w73, y="Vision Good Range") -> (x-y=w72:dbl)
        n52 = call "Label Targets2.vi"("Score Threshold"="Score Threshold", "Targets"=w102, "Image in"=w60) -> ("Image out"=→"Original Image":T2)  [unwired: 8 in]
        n53 = Unbundle(w79) -> (w65:dbl, w67:dbl)
        n54 = Subtract(x=w65, y="Vision Scaling") -> (x-y=w63:dbl)
        n55 = In Range and Coerce(upper limit=w71, x=w63, lower limit=w72) -> (In Range?=→"VISION GOOD":bool)  [unwired: 1 out]
        n56 = Bundle(w63, w67) -> (→"Found Targets":cluster{dbl, dbl})  [unwired: 1 in]
        n57 = call-poly <vilib>:"NT Write Value.vi"("Numeric"=w78, "Name"="Distance") -> ()  [unwired: 9 in, 1 out]
        n58 = feedback-in #1(w65) -> ()
        n59 = feedback #1() -> (w69:dbl)  [unwired: 1 in]
        n60 = call-poly <vilib>:"NT Write Value.vi"("Numeric"=w63, "Name"="Scaled Vision X") -> ()  [unwired: 9 in, 1 out]
        n61 = call-poly <vilib>:"NT Write Value.vi"("Numeric"=w67, "Name"="Vision Y") -> ()  [unwired: 9 in, 1 out]
        n62 = call-poly <vilib>:"NT Write Value.vi"("Numeric"=w69, "Name"="Vision X") -> ()  [unwired: 9 in, 1 out]
        "fps" <- w106
        "Highest Avg Score" <- w99
      }
    }
  }
  n63 = register-events(refnum<vi> refnum, w6) -> (reference out=w26:refnum<event-registration>, error out=w25:errorcluster)  [unwired: 2 in]
  n64 = property class="VI"() -> ("Panel"=w29:refnum<vi>)  [unwired: 2 in, 2 out]
  n65 = while {
    tunnel: w18 -> [w152]
    tunnel: w13 -> [w150]
    tunnel: [w148] -> _
    tunnel: u32 1000 ("milliseconds to wait") -> [w147]
    tunnel: w6 -> [w140]
    i -> [w148]
    stop <- FALSE stop-if-true
    n66 = local read "Rec Mode"() -> (w143:enum32{"Stop", "Record", "Playback"})
    n67 = Wait on Notification(notifier=w150, timeout in ms (-1)=w147) -> (notification=w149:string, timed out?=w145:bool)  [unwired: 2 in, 2 out]
    n68 = Equal?(x=w143, y=u16 2 ("Rec Mode")) -> (x = y?=w144:bool)
    n69 = Compound Arithmetic op=OR(invert w145, w144) -> (w146:bool)
    n70 = case shown="True" w146 {
      tunnel: w152 -> [_ w156]
      tunnel: w149 -> [_ w155]
      tunnel: "Dashboard" -> [_ w154]
      tunnel: w140 -> [_ w153]
      frame False {
      }
      frame True {
        n71 = call <vilib>:"Bind Controls to SmartDashboard.vi"("RPC ref"=w153, "Client Name"=w154, "Bound Control Refs"=w156, "Server IP Address"=w155) -> ()  [unwired: 8 in]
      }
    }
  }
  n72 = vi-ref "Playback Controls.vi"() -> (w27:refnum<vi>)
  n73 = call "Initialize Camera and CheckList.vi"("ListBox in"=w15) -> ("Cluster"=w33:cluster{"value":i32, "value":i32, "index":i32}, "Array"=w34:cluster{string[]}[], "File Refnum"=w32:T22)  [unwired: 8 in]
  n74 = property class="Pnl"(reference=w29) -> ("Panes[]"=w30:refnum<vi>[])  [unwired: 1 in, 2 out]
  n75 = property on="Camera Settings" class="Clust (strict)"("Val(Sgnl)"=w33) -> ()  [unwired: 2 in, 2 out]
  n76 = Index Array(array=w30) -> (element=w28:refnum<vi>)  [unwired: 1 in]
  n77 = while {
    tunnel: [w168] -> _
    tunnel: w13 -> [w162]
    tunnel: w12 -> [w161]
    tunnel: w11 -> [w157]
    i -> [w168]
    stop <- FALSE stop-if-true
    n78 = local read "Vision"() -> (w159:u16)
    n79 = call <vilib>:"WPI_DashboardUpdateNames.vi"("Controls on Tab"=w161) -> ()  [unwired: 11 in]
    n80 = call <vilib>:"WPI_DashboardRetrieveStatusInfo.vi"("Vision"=w159, "Binding Refnum"=w162, "Window Mode Notifier"=w157, "TCP Cnx"="TCP") -> ("Power and Errors"=w163:T23, "Robot Metrics"=w166:T24, "Status Info"=w167:T25, "Control Info"=w164:T26, "Robot Mode"=w160:T13, "Process?"=w165:bool)  [unwired: 2 in]
    "Mode" <- w160
    n81 = case shown="True" w165 {
      tunnel: w167 -> [_ w238]
      tunnel: w166 -> [_ w237]
      tunnel: w164 -> [_ w236]
      tunnel: w163 -> [_ w235]
      tunnel: w160 -> [_ _]
      frame False {
        n82 = Wait (ms)(milliseconds to wait=u32 20) -> ()  [unwired: 1 out]
      }
      frame True {
        # "Get Data from robot"
        # "Send data to robot"
        # "swap motors to match\ncharts and include battery"
        n83 = Unbundle By Name(w236) -> ("Joystick Values"=w225:T27)  [unwired: 1 out]
        n84 = Unbundle By Name(w235) -> ("Camera Addr"=→"Camera IP":string)  [unwired: 1 out]
        n85 = Unbundle By Name(w237) -> ()  [unwired: 1 out]
        n86 = Unbundle By Name(w238) -> ("Battery V"=w226:dbl)  [unwired: 1 out]
        n87 = Index Array(array=w225) -> (element #1=w224:T28, element #2=w219:T28)  [unwired: 2 in]
        n88 = call "Prepare Joystick Data for Displays.vi"("Joystick Values"=w219) -> ("Buttons"=→"JS2 Buttons":T29, "Z Axis"=→"JS2 Z":dbl, "Cartesian Data"=→"JS2 Graph":cluster{"X axis":dbl, "X axis":dbl}[])  [unwired: 8 in]
        n89 = call "Prepare Joystick Data for Displays.vi"("Joystick Values"=w224) -> ("Buttons"=→"JS1 Buttons":T29, "Z Axis"=→"JS1 Z":dbl, "Cartesian Data"=→"JS1 Graph":cluster{"X axis":dbl, "X axis":dbl}[])  [unwired: 8 in]
        n90 = call-poly <vilib>:"NT Read Value.vi"("Name"="RobotDrive Motors") -> ("Numeric Array"=w214:dbl[])  [unwired: 9 in, 1 out]
        n91 = Index Array(array=w214, index #1=1, index #4=0) -> (element #1=w230:dbl, element #2=w231:dbl, element #3=w229:dbl, element #4=w234:dbl)  [unwired: 2 in]
        n92 = Bundle("Numeric"=w229, "Numeric"=w230) -> (→"MotorChart R" →"MotorSliders R":cluster{"Numeric":dbl, "Numeric":dbl})  [unwired: 1 in]
        n93 = Bundle("Numeric"=w231, "Numeric"=w234, "Battery V"=w226) -> (→"MotorChart L" →"MotorSliders L":T10)  [unwired: 1 in]
        n94 = call-poly <vilib>:"NT Read Value.vi"("Name"="WHEELS GOOD") -> ("Boolean"=→"Wheels Good":bool)  [unwired: 9 in, 1 out]
        n95 = call-poly <vilib>:"NT Read Value.vi"("Name"="Encoder Distance") -> ("Numeric"=→"Encoder Distance":dbl)  [unwired: 9 in, 1 out]
        n96 = call-poly <vilib>:"NT Read Value.vi"("Name"="Arm Angle") -> ("Numeric"=→"Arm Angle":dbl)  [unwired: 9 in, 1 out]
        n97 = call-poly <vilib>:"NT Read Value.vi"("Name"="Gyro Angle") -> ("Numeric"=→"Gyro" →"Gyro":dbl)  [unwired: 9 in, 1 out]
        n98 = call-poly <vilib>:"NT Read Value.vi"("Name"="Encoder Gyro") -> ("Numeric"=→"Encoder Gyro":dbl)  [unwired: 9 in, 1 out]
        n99 = call-poly <vilib>:"NT Read Value.vi"("Name"="ARM GOOD") -> ("Boolean"=→"Arm Good":bool)  [unwired: 9 in, 1 out]
        n100 = call-poly <vilib>:"NT Read Value.vi"("Name"="Arm Angle Setpoint") -> ("Numeric"=→"Angle SP":dbl)  [unwired: 9 in, 1 out]
        n101 = call-poly <vilib>:"NT Read Value.vi"("Name"="Shooter RPM Setpoint") -> ("Numeric"=→"RPM SP":dbl)  [unwired: 9 in, 1 out]
        n102 = call-poly <vilib>:"NT Read Value.vi"("Name"="Wheel RPM L") -> ("Numeric"=→"RPM L":dbl)  [unwired: 9 in, 1 out]
        n103 = call-poly <vilib>:"NT Read Value.vi"("Name"="Wheel RPM R") -> ("Numeric"=→"RPM R":dbl)  [unwired: 9 in, 1 out]
        n104 = call-poly <vilib>:"NT Read Value.vi"("Name"="Intake ON") -> ("Boolean"=→"Intake":bool)  [unwired: 9 in, 1 out]
        n105 = call-poly <vilib>:"NT Read Value.vi"("Name"="Shooter ON") -> ("Boolean"=→"Shooter":bool)  [unwired: 9 in, 1 out]
        n106 = call-poly <vilib>:"NT Read Value.vi"("Name"="Ball Holder OR") -> ("Boolean"=→"Ball Holder OR":bool)  [unwired: 9 in, 1 out]
        n107 = call-poly <vilib>:"NT Write Value.vi"("Numeric"="OW Arm Angle", "Name"="D4 Arm Angle") -> ()  [unwired: 9 in, 1 out]
        n108 = call-poly <vilib>:"NT Write Value.vi"("Numeric"="D4 Wheel Speed", "Name"="D4 Wheel Speed") -> ()  [unwired: 9 in, 1 out]
        n109 = call-poly <vilib>:"NT Write Value.vi"("Numeric"="Auto Selection", "Name"="Auto") -> ()  [unwired: 9 in, 1 out]
        n110 = call-poly <vilib>:"NT Write Value.vi"("Numeric"="Fender Wheel Speed", "Name"="Fender Wheel Speed") -> ()  [unwired: 9 in, 1 out]
        n111 = call-poly <vilib>:"NT Write Value.vi"("Numeric"="148 Arm Angle", "Name"="Fender Arm Angle") -> ()  [unwired: 9 in, 1 out]
        n112 = local read "Wheels Good"() -> (w185:bool)
        n113 = local read "VISION GOOD"() -> (w186:bool)
        n114 = local read "Arm Good"() -> (w183:bool)
        n115 = call-poly <vilib>:"NT Write Value.vi"("Boolean"="Gyro Reset", "Name"="Gyro Reset") -> ()  [unwired: 9 in, 1 out]
        n116 = And(x=w185, y=w186) -> (x .and. y?=w184:bool)
        n117 = And(x=w183, y=w184) -> (x .and. y?=→"Boolean" →"Boolean 2" →"Boolean 4" →"Boolean 3":bool)
      }
    }
  }
  n118 = control-ref of="Test Tree"() -> (w31:refnum<vi>)
  n119 = while {
    tunnel: w34 -> [w250]
    shift-right: [w249] -> _
    shift-left: w32 -> [w248]
    tunnel: [w247] -> _
    tunnel: w31 -> [w246]
    tunnel: w27 -> [w245]
    tunnel: w26 -> [w244]
    tunnel: w25 -> [_]
    tunnel: w21 -> [w243]
    tunnel: w6 -> [w242]
    tunnel: w5 -> [w241]
    shift-right: [w240] -> _
    shift-left: _ -> [w239]
    i -> [w247]
    stop <- FALSE stop-if-true
    n120 = event shown="[23] \"Tree\": Double Click" {
      selector: w244 -> [_ _ _ _ _ _ _ _ _ _ _ _ _ _ _ _ _ _ _ _ _ _ _ _]
      dyn-events: [_ _ _ _ _ _ _ _ _ _ _ _ _ _ _ _ _ _ w557 _ _ _ _ _] -> _
      timeout: u32 60 ("milliseconds to wait") -> [_ _ _ _ _ _ _ _ _ _ _ _ _ _ _ _ _ _ _ _ _ _ _ _]
      tunnel: w246 -> [w263 _ _ _ _ _ _ _ _ _ _ _ _ _ _ _ _ _ _ _ _ _ _ _]
      tunnel: "Test Tree" -> [_ _ _ _ _ _ _ _ _ _ _ _ _ w522 w531 w534 w539 w548 _ _ _ _ _ _]
      tunnel: w250 -> [_ w301 _ _ _ _ _ _ _ _ _ w484 w515 _ _ _ _ _ _ _ _ _ _ _]
      tunnel: [w260 w300 w404 w410 w420 w424 w430 w442 w450 w456 w469 w483 w508 w521 w529 w533 w538 w547 w559 w575 w577 w585 w596 w601] -> w249
      tunnel: w248 -> [w260 w300 w404 w410 w420 w424 w430 w442 w450 w456 w469 w482 w508 w521 w529 w533 w538 w547 w559 w575 w577 w585 w596 w601]
      tunnel: w245 -> [_ _ _ _ _ _ _ _ _ _ _ _ _ _ _ _ _ _ w560 _ w580 _ _ _]
      tunnel: w243 -> [_ _ _ _ _ _ _ _ _ _ _ _ _ _ _ _ _ _ w555 _ _ _ _ _]
      tunnel: w242 -> [_ _ _ _ _ _ _ _ _ _ _ _ _ _ _ _ _ _ w553 _ _ _ _ _]
      tunnel: w241 -> [w255 _ _ _ _ _ w428 _ _ _ _ _ _ _ _ _ _ _ _ _ _ _ _ _]
      tunnel: [w254 w299 w403 w409 w419 w425 w426 w436 w447 w455 w468 w481 w507 w520 w528 w532 w537 w546 w552 w573 w576 w581 w589 w602] -> w240
      tunnel: w239 -> [w254 w299 w403 w409 w419 w425 w426 _ _ w455 w468 w481 w507 w520 w528 w532 w537 w546 w552 w573 w576 w581 w589 w602]
      event Timeout {
        n121 = event-data() -> ()  [unwired: 1 in, 1 out]
        n122 = local read "Mode"() -> (w257:T13)
        n123 = call <vilib>:"NT Read String.vi"("Name"="/TestMode/TestName") -> ("String"=w266:string)  [unwired: 9 in, 1 out]
        n124 = case shown="\"Test\"" "Dashboard Tab" {
          tunnel: w263 -> [_ w277 _ _]
          tunnel: "/TestMode/Automatic/" ("Name Pattern") -> [_ w276 _ _]
          tunnel: T30 [{"Operation"=enum."Clear", "Color Box"=14013909}, {"Operation"=enum."Clear", "Color Box"=14013909}, {"Operation"=enum."Clear", "Color Box"=14013909}, {"Operation"=enum."Clear", "Color Box"=14013909}, {"Operation"=enum."Update", "Color Box"=14013909}, {"Operation"=enum."Update", "Color Box"=16777215}, {"Operation"=enum."Clear", "Color Box"=14013909}, {"Operation"=enum."Clear", "Color Box"=14013909}, {"Operation"=enum."Clear", "Color Box"=14013909}] -> [_ w269 _ w286]
          tunnel: w257 -> [_ w268 _ w285]
          tunnel: u32[] [15790320, 15790320, 15790320, 15790320, 16777215, 16777215, 15790320, 15790320, 15790320] -> [_ _ _ w291]
          tunnel: w255 -> [_ _ _ w279]
          frame "Driver", Default {
          }
          frame "Test" {
            w275 = -2 ("Active Item:Row Number")
            n125 = Index Array(array=w269, index=w268) -> (element=w270:T34)
            n126 = Unbundle(w270) -> ("Operation"=w271:enum16{"Update", "Clear"}, "Color Box"=w272:u32)
            n127 = call <vilib>:"NT Read and Format Entries as Tree.vi"("Operation"=w271, "Name Pattern"=w276, "Tree Refnum"=w277) -> ()  [unwired: 7 in, 2 out]
            n128 = property on="Test Tree" class="Tree (strict)"("Active Item Row Number"=w275, "ActiveColNum"=w275, "CellBG"=w272, "Active Item Row Number"=-1 ("Active Item:Row Number"), "CellBG"=u32 5789784 ("Color Box")) -> ()  [unwired: 2 in, 2 out]
          }
          frame "Variables" {
            n129 = control-ref of="Tree"() -> (w278:refnum<vi>)
            n130 = call <vilib>:"NT Read and Format Entries as Tree.vi"("Tree Refnum"=w278) -> ()  [unwired: 9 in, 2 out]
          }
          frame "Commands" {
            w287 = u32 5789784 ("Color Box")
            w288 = T35 {"Row"=-1, "Column"=-2} ("Active Cell:Active Cell")
            w290 = T35 {"Row"=-2, "Column"=-2} ("Active Cell:Active Cell")
            n131 = Index Array(array=w291, index=w285) -> (element=w289:u32)
            n132 = Index Array(array=w286, index=w285) -> (element=w284:T34)
            n133 = Unbundle(w284) -> ("Operation"=w283:enum16{"Update", "Clear"})  [unwired: 1 out]
            n134 = local read "Command Selection"() -> (w282:i32)
            n135 = property on="Command Selection" class="MCListbox (strict)"("ActiveCell"=w290, "CellBG"=w289, "ActiveCell"=w288, "CellBG"=w287) -> ()  [unwired: 2 in, 2 out]
            n136 = call <vilib>:"WPI_DashboardUpdate RPC Info.vi"("Operation"=w283) -> ("update"=w281:bool, "commands"=w280:string[][])  [unwired: 9 in]
            n137 = property on="Command Selection" class="MCListbox (strict)"("ItemNames"=w280) -> ()  [unwired: 2 in, 2 out]
            n138 = property on="Command Params" class="Tbl (strict)"("Active Cell"=w290, "Cell BG Color"=w289, "Active Cell"=w288, "Cell BG Color"=w287) -> ()  [unwired: 2 in, 2 out]
            n139 = call <vilib>:"WPI_DashboardUpdate Command Params.vi"("Update"=w281, "NewVal"=w282, "Commands"=w280, "Param Tbl"=w279) -> ()  [unwired: 7 in, 1 out]
          }
        }
        n140 = case shown="\"\"" w266 {
          tunnel: "/TestMode/TestProgress" ("Name") -> [w293 _]
          tunnel: "/TestMode/TestProgressText" ("Name") -> [w292 _]
          frame Default {
            n141 = call <vilib>:"NT Read Number.vi"("Name"=w293) -> ("Numeric"=w294:dbl)  [unwired: 9 in, 1 out]
            n142 = call <vilib>:"NT Read String.vi"("Name"=w292) -> ("String"=w295:string)  [unwired: 9 in, 1 out]
            n143 = Bundle("Numeric"=w294, "String"=w295) -> (→"Progress":cluster{"Numeric":dbl, "String":string})  [unwired: 1 in]
          }
          frame "" {
            n144 = property on="Progress" class="Clust (strict)"("Visible"=FALSE) -> ()  [unwired: 2 in, 2 out]
            n145 = local write "Test Name"(u16 0) -> ()
          }
        }
        n146 = call <vilib>:"Connextion Info.vi"() -> ("Connected"=→"NT Connection":bool)  [unwired: 10 in, 1 out]
      }
      event "Test Tree": Value Change {
        # "Show appropriate\ncontrols"
        n147 = event-data() -> ("CtlRef"=w304:refnum<vi>, "NewVal"=w302:string)  [unwired: 1 in]
        n148 = call <vilib>:"WPI_UtilitiesGetTreeIOName.vi"("NewVal"=w302, "TreeControl in"=w304) -> ("I/O Name"=w305:string)  [unwired: 9 in]
        n149 = case shown="\"Analog Out\", \"Motor\", \"PWM\"" w305 {
          selector: w305 -> [_ w312 _ w334 w343 _]
          tunnel: w302 -> [_ _ w331 w333 _ w350]
          tunnel: w301 -> [_ _ _ _ _ w349]
          frame Default {
            w307 = FALSE ("Visible")
            w306 = FALSE ("Visible")
            n150 = property on="Motor" class="Clust (strict)"("Visible"=w306) -> ()  [unwired: 2 in, 2 out]
            n151 = property on="Test Ring" class="Ring (strict)"("Visible"=w306) -> ()  [unwired: 2 in, 2 out]
            n152 = property on="Rev/Fwd" class="Clust (strict)"("Visible"=w307) -> ()  [unwired: 2 in, 2 out]
            n153 = property on="On/Off" class="Bool (strict)"("Visible"=w307) -> ()  [unwired: 2 in, 2 out]
            n154 = property on="Test Slider" class="Slide (strict)"("Visible"=w307) -> ()  [unwired: 2 in, 2 out]
          }
          frame "Analog Out", "Motor", "PWM" {
            w313 = FALSE ("Visible")
            n155 = case shown="\"Analog Out\"" w312 {
              tunnel: [1.0 ("Value") -1.0 ("Value") 0.0 ("Value")] -> w311
              tunnel: [255.0 ("Value") 1.0 ("Value") 5.0 ("Value")] -> w310
              tunnel: [128.0 ("Value") 0.0 ("Value") 0.0 ("Value")] -> w309
              tunnel: [64.0 ("Value") 0.5 ("Value") 1.0 ("Value")] -> w308
              frame "PWM" {
              }
              frame "Motor", Default {
              }
              frame "Analog Out" {
              }
            }
            n156 = property on="Motor" class="Clust (strict)"("Visible"=TRUE) -> ()  [unwired: 2 in, 2 out]
            n157 = property on="Value" class="Slide (strict)"("Value"=w309, "Scale.Minimum"=w311, "Scale.Maximum"=w310, "Scale.Increment"=w308) -> ()  [unwired: 2 in, 2 out]
            n158 = property on="On/Off" class="Bool (strict)"("Visible"=w313) -> ()  [unwired: 2 in, 2 out]
            n159 = property on="Test Slider" class="Slide (strict)"("Visible"=w313) -> ()  [unwired: 2 in, 2 out]
            n160 = property on="Test Ring" class="Ring (strict)"("Visible"=w313) -> ()  [unwired: 2 in, 2 out]
            n161 = property on="Rev/Fwd" class="Clust (strict)"("Visible"=w313) -> ()  [unwired: 2 in, 2 out]
          }
          frame "Servo" {
            w329 = FALSE ("Visible")
            n162 = call <vilib>:"NT Read Number.vi"("Name"=w331) -> ("Numeric"=w330:dbl)  [unwired: 9 in, 1 out]
            n163 = property on="Test Slider" class="Slide (strict)"("Visible"=TRUE, "Scale.Maximum"=170.0 ("Scale.Range:Maximum")) -> ()  [unwired: 2 in, 2 out]
            n164 = local write "Test Slider"(w330) -> ()
            n165 = property on="Motor" class="Clust (strict)"("Visible"=w329) -> ()  [unwired: 2 in, 2 out]
            n166 = property on="Rev/Fwd" class="Clust (strict)"("Visible"=w329) -> ()  [unwired: 2 in, 2 out]
            n167 = property on="On/Off" class="Bool (strict)"("Visible"=w329) -> ()  [unwired: 2 in, 2 out]
            n168 = property on="Test Ring" class="Ring (strict)"("Visible"=w329) -> ()  [unwired: 2 in, 2 out]
          }
          frame "Relay", "Solenoid" {
            w332 = FALSE ("Visible")
            n169 = property on="Motor" class="Clust (strict)"("Visible"=w332) -> ()  [unwired: 2 in, 2 out]
            n170 = property on="Test Slider" class="Slide (strict)"("Visible"=w332) -> ()  [unwired: 2 in, 2 out]
            n171 = Search and Replace String(input string=w333, search string="/Value  **", replace string="/Direction") -> (result string=w339:string)  [unwired: 5 in, 3 out]
            n172 = property on="Test Ring" class="Ring (strict)"("Visible"=w332) -> ()  [unwired: 2 in, 2 out]
            n173 = call <vilib>:"NT Read String.vi"("Name"=w339) -> ("String"=w337:string)  [unwired: 9 in, 1 out]
            n174 = Equal?(x="Both directions", y=w337) -> (x = y?=w335:bool)
            n175 = Not(x=w335) -> (.not. x?=w336:bool)
            n176 = property on="Rev/Fwd" class="Clust (strict)"("Visible"=w335) -> ()  [unwired: 2 in, 2 out]
            n177 = property on="On/Off" class="Bool (strict)"("Visible"=w336, "Caption.Text"=w334) -> ()  [unwired: 2 in, 2 out]
          }
          frame "Compressor", "Digital Out" {
            w342 = FALSE ("Visible")
            # "Get direction and finish"
            n178 = property on="Motor" class="Clust (strict)"("Visible"=w342) -> ()  [unwired: 2 in, 2 out]
            n179 = property on="Test Slider" class="Slide (strict)"("Visible"=w342) -> ()  [unwired: 2 in, 2 out]
            n180 = property on="Test Ring" class="Ring (strict)"("Visible"=w342) -> ()  [unwired: 2 in, 2 out]
            n181 = property on="On/Off" class="Bool (strict)"("Visible"=TRUE, "Caption.Text"=w343) -> ()  [unwired: 2 in, 2 out]
            n182 = property on="Rev/Fwd" class="Clust (strict)"("Visible"=FALSE) -> ()  [unwired: 2 in, 2 out]
          }
          frame "Camera" {
            n183 = call <vilib>:"Get Last Path Segment.vi"("String in"=w350) -> ("String out"=w351:string)  [unwired: 10 in]
            n184 = property on="On/Off" class="Bool (strict)"("Visible"=FALSE) -> ()  [unwired: 2 in, 2 out]
            n185 = property on="Motor" class="Clust (strict)"("Visible"=FALSE) -> ()  [unwired: 2 in, 2 out]
            n186 = property on="Rev/Fwd" class="Clust (strict)"("Visible"=FALSE) -> ()  [unwired: 2 in, 2 out]
            n187 = case shown="\"White Balance  **\"" w351 {
              tunnel: w350 -> [w357 w366 w375 w384 w393 _ w399]
              tunnel: w349 -> [w355 w363 w372 w381 w390 _ _]
              frame "Size  **" {
                n188 = Index Array(array=w355) -> (element=w354:cluster{string[]})  [unwired: 1 in]
                n189 = call <vilib>:"NT Read String.vi"("Name"=w357) -> ("String"=w356:string)  [unwired: 9 in, 1 out]
                n190 = Unbundle(w354) -> (w352:string[])
                n191 = Match First String(2:w352, 3:w356) -> (0:w353:i32)  [unwired: 1 out]
                n192 = property on="Test Ring" class="Ring (strict)"("Value"=w353, "Strings []"=w352) -> ()  [unwired: 2 in, 2 out]
                n193 = property on="Test Ring" class="Ring (strict)"("Visible"=TRUE) -> ()  [unwired: 2 in, 2 out]
                n194 = property on="Test Slider" class="Slide (strict)"("Visible"=FALSE) -> ()  [unwired: 2 in, 2 out]
              }
              frame "White Balance  **" {
                n195 = Index Array(array=w363, index=1) -> (element=w364:cluster{string[]})
                n196 = call <vilib>:"NT Read String.vi"("Name"=w366) -> ("String"=w365:string)  [unwired: 9 in, 1 out]
                n197 = Unbundle(w364) -> (w361:string[])
                n198 = Match First String(2:w361, 3:w365) -> (0:w360:i32)  [unwired: 1 out]
                n199 = property on="Test Ring" class="Ring (strict)"("Value"=w360, "Strings []"=w361) -> ()  [unwired: 2 in, 2 out]
                n200 = property on="Test Ring" class="Ring (strict)"("Visible"=TRUE) -> ()  [unwired: 2 in, 2 out]
                n201 = property on="Test Slider" class="Slide (strict)"("Visible"=FALSE) -> ()  [unwired: 2 in, 2 out]
              }
              frame "Exposure  **" {
                n202 = Index Array(array=w372, index=2) -> (element=w373:cluster{string[]})
                n203 = call <vilib>:"NT Read String.vi"("Name"=w375) -> ("String"=w374:string)  [unwired: 9 in, 1 out]
                n204 = Unbundle(w373) -> (w369:string[])
                n205 = Match First String(2:w369, 3:w374) -> (0:w370:i32)  [unwired: 1 out]
                n206 = property on="Test Ring" class="Ring (strict)"("Value"=w370, "Strings []"=w369) -> ()  [unwired: 2 in, 2 out]
                n207 = property on="Test Ring" class="Ring (strict)"("Visible"=TRUE) -> ()  [unwired: 2 in, 2 out]
                n208 = property on="Test Slider" class="Slide (strict)"("Visible"=FALSE) -> ()  [unwired: 2 in, 2 out]
              }
              frame "Exposure Priority  **" {
                n209 = Index Array(array=w381, index=3) -> (element=w382:cluster{string[]})
                n210 = call <vilib>:"NT Read String.vi"("Name"=w384) -> ("String"=w383:string)  [unwired: 9 in, 1 out]
                n211 = Unbundle(w382) -> (w378:string[])
                n212 = Match First String(2:w378, 3:w383) -> (0:w379:i32)  [unwired: 1 out]
                n213 = property on="Test Ring" class="Ring (strict)"("Value"=w379, "Strings []"=w378) -> ()  [unwired: 2 in, 2 out]
                n214 = property on="Test Ring" class="Ring (strict)"("Visible"=TRUE) -> ()  [unwired: 2 in, 2 out]
                n215 = property on="Test Slider" class="Slide (strict)"("Visible"=FALSE) -> ()  [unwired: 2 in, 2 out]
              }
              frame "Color Enable  **" {
                n216 = Index Array(array=w390, index=4) -> (element=w391:cluster{string[]})
                n217 = call <vilib>:"NT Read String.vi"("Name"=w393) -> ("String"=w392:string)  [unwired: 9 in, 1 out]
                n218 = Unbundle(w391) -> (w387:string[])
                n219 = Match First String(2:w387, 3:w392) -> (0:w388:i32)  [unwired: 1 out]
                n220 = property on="Test Ring" class="Ring (strict)"("Value"=w388, "Strings []"=w387) -> ()  [unwired: 2 in, 2 out]
                n221 = property on="Test Ring" class="Ring (strict)"("Visible"=TRUE) -> ()  [unwired: 2 in, 2 out]
                n222 = property on="Test Slider" class="Slide (strict)"("Visible"=FALSE) -> ()  [unwired: 2 in, 2 out]
              }
              frame Default {
                n223 = property on="Test Ring" class="Ring (strict)"("Visible"=FALSE) -> ()  [unwired: 2 in, 2 out]
                n224 = property on="Test Slider" class="Slide (strict)"("Visible"=FALSE) -> ()  [unwired: 2 in, 2 out]
              }
              frame "Brightness  **", "Color Level  **", "Compression  **", "FPS  **", "Sharpness  **" {
                n225 = call <vilib>:"NT Read Number.vi"("Name"=w399) -> ("Numeric"=w398:dbl)  [unwired: 9 in, 1 out]
                n226 = local write "Test Slider"(w398) -> ()
                n227 = property on="Test Slider" class="Slide (strict)"("Visible"=TRUE, "Scale.Maximum"=100.0 ("Scale.Range:Maximum")) -> ()  [unwired: 2 in, 2 out]
                n228 = property on="Test Ring" class="Ring (strict)"("Visible"=FALSE) -> ()  [unwired: 2 in, 2 out]
              }
            }
          }
        }
        n229 = property on="Progress" class="Clust (strict)"("Visible"=FALSE) -> ()  [unwired: 2 in, 2 out]
      }
      event "Test Name": Mouse Enter {
        # "Populate the ring with the list of tests"
        n230 = event-data() -> ()  [unwired: 1 in, 1 out]
        n231 = call <vilib>:"NT Read String Array.vi"("Name"="/TestMode/TestList") -> ("String Array"=w408:string[])  [unwired: 9 in, 1 out]
        n232 = Build Array (concatenate)("Select the test to run...", w408) -> (w407:string[])
        n233 = property on="Test Name" class="Ring (strict)"("Strings []"=w407) -> ()  [unwired: 2 in, 2 out]
      }
      event "Test Name": Value Change {
        w411 = FALSE ("Visible")
        # "Tell the robot the test name to run"
        n234 = event-data() -> ("NewVal"=w415:u16)  [unwired: 1 in]
        n235 = property on="Test Name" class="Ring (strict)"() -> ("Strings []"=w416:string[])  [unwired: 2 in, 2 out]
        n236 = local write "Progress"(T14 {"Test Progress"=0, "Test Progress Text"=""} ("Progress")) -> ()
        n237 = Index Array(array=w416, index=w415) -> (element=w414:string)
        n238 = call <vilib>:"NT Write String.vi"("String"=w414, "Name"="/TestMode/TestName") -> ()  [unwired: 9 in, 1 out]
        n239 = property on="Progress" class="Clust (strict)"("Visible"=TRUE) -> ()  [unwired: 2 in, 2 out]
        n240 = property on="Motor" class="Clust (strict)"("Visible"=w411) -> ()  [unwired: 2 in, 2 out]
        n241 = property on="Test Slider" class="Slide (strict)"("Visible"=w411) -> ()  [unwired: 2 in, 2 out]
        n242 = property on="On/Off" class="Bool (strict)"("Visible"=w411) -> ()  [unwired: 2 in, 2 out]
        n243 = property on="Rev/Fwd" class="Clust (strict)"("Visible"=w411) -> ()  [unwired: 2 in, 2 out]
        n244 = property on="Test Ring" class="Ring (strict)"("Visible"=w411) -> ()  [unwired: 2 in, 2 out]
      }
      event "Select Auto": Mouse Enter {
        # "Populate the combo box with the list of autonomous options"
        n245 = event-data() -> ()  [unwired: 1 in, 1 out]
        n246 = call <vilib>:"NT Read String Array.vi"("Name"="Auto List") -> ("String Array"=w418:string[])  [unwired: 9 in, 1 out]
        n247 = property on="Select Auto" class="CmbBox"("Strings[]"=w418) -> ()  [unwired: 2 in, 2 out]
      }
      event "Select Auto": Value Change {
        # "User modified the Auto Selection. Write to NT variable so robot knows."
        n248 = event-data() -> ("NewVal"=w422:string)  [unwired: 1 in]
        n249 = call <vilib>:"NT Write String.vi"("String"=w422, "Name"="Auto Selector") -> ()  [unwired: 9 in, 1 out]
      }
      event "Command Selection": Value Change {
        # "Get the params and show in table"
        n250 = event-data() -> ("NewVal"=w429:i32)  [unwired: 1 in]
        n251 = property on="Command Selection" class="MCListbox (strict)"() -> ("ItemNames"=w427:string[][])  [unwired: 2 in, 2 out]
        n252 = call <vilib>:"WPI_DashboardUpdate Command Params.vi"("NewVal"=w429, "Commands"=w427, "Param Tbl"=w428) -> ()  [unwired: 8 in, 1 out]
      }
      event "Execute Command": Value Change {
        # "Started one, Unique ID holds\nresponse"
        n253 = event-data() -> ()  [unwired: 1 in, 1 out]
        n254 = property on="Command Selection" class="MCListbox (strict)"() -> ("ItemNames"=w441:string[][])  [unwired: 2 in, 2 out]
        n255 = Index Array(array=w441, index (row)="Command Selection", index (col)=0) -> (element=w439:string)
        n256 = call <vilib>:"Invoke Commands.vi"("Command Params"="Command Params", "Function Name"=w439) -> ("Params"=w435:u8, "Started"=w434:bool)  [unwired: 7 in, 1 out]
        n257 = Array Subset(array="Command Params", length (row)=w435) -> (w436:string[][])  [unwired: 3 in]
        n258 = Select(t="Executing" ("Cmd Status"), s=w434, f="" ("Cmd Status")) -> (s? t:f=→"Cmd Status":string)
      }
      event "Command Selection": Double Click {
        n259 = event-data() -> ("Row"=w451:i32)  [unwired: 1 in]
        n260 = property on="Command Selection" class="MCListbox (strict)"() -> ("ItemNames"=w454:string[][])  [unwired: 2 in, 2 out]
        n261 = local read "Command Params"() -> (w449:string[][])
        n262 = Index Array(array=w454, index (row)=w451, index (col)=0) -> (element=w452:string)
        n263 = call <vilib>:"Invoke Commands.vi"("Command Params"=w449, "Function Name"=w452) -> ("Params"=w448:u8, "Started"=w443:bool)  [unwired: 7 in, 1 out]
        n264 = Array Subset(array=w449, length (row)=w448) -> (w447:string[][])  [unwired: 3 in]
        n265 = Select(t="Executing" ("Cmd Status"), s=w443, f="" ("Cmd Status")) -> (s? t:f=w444:string)
        n266 = local write "Cmd Status"(w444) -> ()
      }
      event "CheckList": Double Click {
        # "Shift clears all"
        # "Update symbols on the listbox"
        n267 = event-data() -> ("PlatMods.Shift"=w457:bool, "Row"=w459:i32)  [unwired: 1 in]
        n268 = case shown="True" w457 {
          tunnel: w459 -> [w463 _]
          tunnel: 1 -> [w462 _]
          frame False {
            n269 = property on="CheckList" class="LstBox (strict)"() -> ("Item Symbols"=w461:i32[])  [unwired: 2 in, 2 out]
            n270 = Replace Array Subset(array=w461, new element=w462, index=w463) -> (w460:i32[])
            n271 = property on="CheckList" class="LstBox (strict)"("Item Symbols"=w460) -> ()  [unwired: 2 in, 2 out]
          }
          frame True {
            w464 = 0 ("Top Row")
            n272 = property on="CheckList" class="LstBox (strict)"() -> ("Number of Rows"=w466:u32)  [unwired: 2 in, 2 out]
            n273 = Initialize Array(0, w466) -> (w465:i32[])
            n274 = property on="CheckList" class="LstBox (strict)"("Top Row"=w464, "Value"=w464, "Item Symbols"=w465) -> ()  [unwired: 2 in, 2 out]
          }
        }
      }
      event "CheckList": Key Down {
        # "Update symbols on the listbox\nLeft and right keys check and uncheck"
        n275 = event-data() -> ("VKey"=w471:T31)  [unwired: 1 in]
        n276 = case shown="\"Left\", \"Right\"" w471 {
          selector: w471 -> [w476 _]
          tunnel: eventvkey."Left" ("VKey") -> [w474 _]
          frame "Left", "Right" {
            n277 = Equal?(x=w474, y=w476) -> (x = y?=w475:bool)
            n278 = Select(t=0, s=w475, f=1) -> (s? t:f=w477:i32)
            n279 = property on="CheckList" class="LstBox (strict)"() -> ("Item Symbols"=w480:i32[])  [unwired: 2 in, 2 out]
            n280 = Replace Array Subset(array=w480, new element=w477, index="CheckList") -> (w479:i32[])
            n281 = property on="CheckList" class="LstBox (strict)"("Item Symbols"=w479) -> ()  [unwired: 2 in, 2 out]
          }
          frame Default {
          }
        }
      }
      event "DB Camera Config": Value Change {
        # "Show or hide the cluster of controls, store in ini file"
        n282 = event-data() -> ("NewVal"=w485:bool)  [unwired: 1 in]
        n283 = case shown="False" w485 {
          tunnel: w484 -> [w494 _]
          tunnel: [w487 w505] -> w483
          tunnel: w482 -> [w486 w505]
          frame False {
            w501 = "Camera"
            w504 = FALSE ("Visible")
            n284 = local read "Camera Settings"() -> (w493:T9)
            n285 = Index Array(array=w494) -> (element=w497:cluster{string[]})  [unwired: 1 in]
            n286 = Unbundle(w493) -> ("Frame Rate"=w492:i32, "Compression"=w491:i32, "Size"=w495:u16)
            n287 = Unbundle(w497) -> (w496:string[])
            n288 = Index Array(array=w496, index=w495) -> (element=w490:string)
            n289 = call-poly <vilib>:"Write Key.vi"("section"=w501, "value"=w490, "key"="Size", "refnum"=w486) -> ("refnum out"=w503:T22)  [unwired: 2 in, 5 out]
            n290 = call-poly <vilib>:"Write Key.vi"("section"=w501, "value"=w492, "key"="FrameRate", "refnum"=w503) -> ("refnum out"=w502:T22)  [unwired: 1 in, 6 out]
            n291 = property on="Camera Settings" class="Clust (strict)"("Visible"=w504) -> ()  [unwired: 2 in, 2 out]
            n292 = local write "DB Camera Config"(w504) -> ()
            n293 = call-poly <vilib>:"Write Key.vi"("section"=w501, "value"=w491, "key"="Compression", "refnum"=w502) -> ("refnum out"=w488:T22)  [unwired: 1 in, 6 out]
            n294 = call <vilib>:"Close Config Data.vi"("refnum"=w488) -> ("file path"=w489:path)  [unwired: 2 in, 8 out]
            n295 = call <vilib>:"Open Config Data.vi"("configuration file path"=w489) -> ("refnum"=w487:T22)  [unwired: 8 in, 2 out]
          }
          frame True {
            n296 = property on="Camera Settings" class="Clust (strict)"("Visible"=TRUE) -> ()  [unwired: 2 in, 2 out]
          }
        }
      }
      event "Camera Settings": Value Change {
        # "Update summary string when any elements of DB camera change"
        n297 = event-data() -> ("NewVal"=w519:T9)  [unwired: 1 in]
        n298 = Index Array(array=w515) -> (element=w514:cluster{string[]})  [unwired: 1 in]
        n299 = Unbundle(w519) -> ("Frame Rate"=w510:i32, "Compression"=w509:i32, "Size"=w512:u16)
        n300 = Unbundle(w514) -> (w513:string[])
        n301 = Index Array(array=w513, index=w512) -> (element=w511:string)
        n302 = Format Into String(format string="%s   %dfps   %d%%", w511, w510, w509) -> (resulting string=w516:string)  [unwired: 2 in, 1 out]
        n303 = Build Array(w516) -> (w517:string[])
        n304 = property on="DB Camera Config" class="Bool (strict)"("Strings [4]"=w517) -> ()  [unwired: 2 in, 2 out]
      }
      event "Motor.Enable": Value Change {
        # "When the test mode otor enable helper is set, update that\ntree row item's value"
        n305 = event-data() -> ("NewVal"=w526:bool)  [unwired: 1 in]
        n306 = Unbundle("Motor") -> ("Value"=w525:dbl)  [unwired: 1 out]
        n307 = Select(t=w525, s=w526, f=0.0) -> (s? t:f=w523:dbl)
        n308 = call <vilib>:"NT Write Number.vi"("Numeric"=w523, "Name"=w522) -> ()  [unwired: 9 in, 1 out]
      }
      event "Test Slider": Value Change {
        # "When the test mode slider helper is set, update that\ntree row item's value"
        n309 = event-data() -> ("NewVal"=w530:dbl)  [unwired: 1 in]
        n310 = call <vilib>:"NT Write Number.vi"("Numeric"=w530, "Name"=w531) -> ()  [unwired: 9 in, 1 out]
      }
      event "On/Off": Value Change {
        # "When the test mode on/off helper value is set, update that\ntree row item's value"
        n311 = event-data() -> ("NewVal"=w536:bool)  [unwired: 1 in]
        n312 = Boolean To (0,1)(Boolean=w536) -> (0, 1=w535:i16)
        n313 = call <vilib>:"NT Write Number.vi"("Numeric"=w535, "Name"=w534) -> ()  [unwired: 9 in, 1 out]
      }
      event "Rev/Fwd": Value Change {
        # "When the test mode helper value for relays is set, update that\ntree row item's value"
        n314 = event-data() -> ("NewVal.Forward"=w545:bool, "NewVal.Reverse"=w544:bool)  [unwired: 1 in]
        n315 = Boolean To (0,1)(Boolean=w545) -> (0, 1=w541:i16)
        n316 = Boolean To (0,1)(Boolean=w544) -> (0, 1=w543:i16)
        n317 = Negate(x=w543) -> (-x=w542:i16)
        n318 = Add(x=w541, y=w542) -> (x+y=w540:i16)
        n319 = call <vilib>:"NT Write Number.vi"("Numeric"=w540, "Name"=w539) -> ()  [unwired: 9 in, 1 out]
      }
      event "Test Ring": Value Change {
        # "When a test mode helper value is selected from the ring,\nset the tree item's variable to the string value"
        n320 = event-data() -> ("NewVal"=w550:u16)  [unwired: 1 in]
        n321 = property on="Test Ring" class="Ring (strict)"() -> ("Strings []"=w551:string[])  [unwired: 2 in, 2 out]
        n322 = Index Array(array=w551, index=w550) -> (element=w549:string)
        n323 = call <vilib>:"NT Write String.vi"("String"=w549, "Name"=w548) -> ()  [unwired: 9 in, 1 out]
      }
      event "Rec Mode": Value Change {
        # "Update globals for recording mode and path to read log from.\nClear when logging and let NetworkTables set path for vision to\nuse."
        n324 = event-data() -> ("NewVal"=w561:enum32{"Stop", "Record", "Playback"})  [unwired: 1 in]
        n325 = global write "WPI_DashboardLogging Global.vi" "Logging Filename"(path "") -> ()
        n326 = global write "WPI_DashboardLogging Global.vi" "Recording"(w561) -> ()
        n327 = case shown="\"Playback\"" w561 {
          tunnel: w560 -> [_ w563 w572]
          tunnel: [_ _ w571] -> w557
          tunnel: [_ _ w570] -> _
          tunnel: w555 -> [_ _ w568]
          tunnel: cluster{i32, i32} {-250, 170} -> [_ _ w567]
          tunnel: [_ _ T32 {"Image Size"=TRUE, "Image Type"=TRUE, "Pixel Value"=TRUE, "ROI Information"=TRUE, "Zoom Factor"=FALSE} ("Image Information Shown:All Elements")] -> _
          tunnel: [_ _ TRUE ("Zoom Factor")] -> _
          tunnel: w553 -> [_ _ w564]
          frame Default {
          }
          frame "Stop", "Record" {
            # "Place Window too"
            n328 = invoke class="VI" method="FP.Close"(reference=w563) -> (reference out=w562:refnum<vi>)  [unwired: 2 in, 2 out]
            n329 = invoke class="VI" method="Abort VI"(reference=w562) -> ()  [unwired: 2 in, 3 out]
          }
          frame "Playback" {
            n330 = call "Open Playback Panel.vi"("Offset"=w567, "DB VI Ref"=w568, "Playback in"=w572) -> ("Playback out"=w569:refnum<vi>)  [unwired: 8 in]
            n331 = register-events(w569, w564) -> (reference out=w571:refnum<event-registration>, error out=w570:errorcluster)  [unwired: 2 in]
          }
        }
        n332 = call <vilib>:"WPI_DashboardNT Log FieldName Cache.vi"("Operation"=enum16{"Lookup/Add", "Index", "Clear"}."Clear") -> ()  [unwired: 8 in, 3 out]
      }
      event Panel Close {
        w574 = enum32{"Stop", "Record", "Playback"}."Stop" ("Rec Mode")
        # "Playback window has been closed, abort"
        n333 = event-data() -> ()  [unwired: 1 in, 4 out]
        n334 = local write "Rec Mode"(w574) -> ()
        n335 = global write "WPI_DashboardLogging Global.vi" "Recording"(w574) -> ()
      }
      event Panel Close {
        # "Abort playback window and ourself"
        n336 = event-data() -> ()  [unwired: 1 in, 4 out]
        n337 = invoke class="VI" method="FP.Close"(reference=w580) -> (reference out=w579:refnum<vi>)  [unwired: 2 in, 2 out]
        n338 = invoke class="VI" method="Abort VI"(reference=w579) -> (error out=w578:errorcluster)  [unwired: 2 in, 2 out]
        n339 = invoke class="VI" method="Abort VI"(error in=w578) -> ()  [unwired: 2 in, 3 out]
      }
      event User Event {
        n340 = event-data() -> ("IDs"=w588:cluster{"RPC field ID":u16, "Unique ID":u16}, "String"=w587:string)  [unwired: 1 in]
        n341 = Bundle("IDs"=w588, "String"=w587) -> (w586:T17)  [unwired: 1 in]
        n342 = call <vilib>:"Retrieve RPC Response.vi"("RPC Response"=w586) -> ("Output"=w583:string[][])  [unwired: 10 in]
        n343 = Build Array (concatenate)(w581, w583) -> (w582:string[][])
        n344 = local write "Command Params"(w582) -> ()
        n345 = local write "Cmd Status"("" ("Cmd Status")) -> ()
      }
      event "Vision": Value Change {
        # "Enable/Disable Compression slider.\nHW USB is hard-coded into the camera"
        n346 = event-data() -> ("NewVal"=w595:u16)  [unwired: 1 in]
        n347 = Equal?(x=w595, y=u32 2 ("milliseconds to wait")) -> (x = y?=w593:bool)
        n348 = Select(t=T33."Disabled and Grayed Out" ("Disabled"), s=w593, f=T33."Enabled" ("Disabled")) -> (s? t:f=w590:T33)
        n349 = property on="Compression" class="Slide (strict)"("DisabledEnum"=w590) -> ()  [unwired: 2 in, 2 out]
      }
      event "Tree": Double Click {
        n350 = event-data() -> ("PlatMods"=w600:T36, "Tag"=w599:string)  [unwired: 1 in]
        n351 = Unbundle(w600) -> ("Shift"=w598:bool)  [unwired: 4 out]
        n352 = Not(x=w598) -> (.not. x?=w597:bool)
        n353 = call <vilib>:"NT Update Persistence.vi"("Persistence"=w597, "Name"=w599) -> ()  [unwired: 9 in, 1 out]
      }
    }
  }
  n354 = while {
    tunnel: w28 -> [w604]
    i -> [w607]
    stop <- FALSE stop-if-true
    n355 = Wait (ms)(milliseconds to wait=u32 100) -> ()  [unwired: 1 out]
    n356 = case shown="\"Playback\"" "Rec Mode" {
      tunnel: w607 -> [_ _ w622]
      tunnel: [u32 2829099 ("Base Color") u32 11141120 ("Target Color") w611] -> w603
      frame "Stop", Default {
        # "Reset the color, extra updates don't cost much"
      }
      frame "Record" {
      }
      frame "Playback" {
        # "Playback"
        n357 = Quotient & Remainder(x=w622, y=u32 50 ("milliseconds to wait")) -> (x-y*floor(x/y)=w618:u32)  [unwired: 1 out]
        n358 = Divide(x=w618, y=u32 50 ("milliseconds to wait")) -> (x/y=w615:dbl)
        n359 = Multiply(x=6.283185307179586, y=w615) -> (x*y=w620:dbl)
        n360 = Sine(x=w620) -> (sin(x)=w619:dbl)
        n361 = Absolute Value(x=w619) -> (abs(x)=w612:dbl)
        n362 = call "Interpolate RGB Color.vi"("Proportion"=w612, "Target Color"=u32 30976, "Base Color"=u32 2829099) -> ("Result Color"=w611:u32)  [unwired: 8 in]
      }
    }
    n363 = property class="Pane"(reference=w604, "PaneColor"=w603) -> ()  [unwired: 1 in, 2 out]
  }
  n364 = disable-structure shown="Disabled" {
    frame Disabled {
      n365 = local write "Dashboard Tab"(T37."Drive" ("Dashboard Tab")) -> ()
    }
    frame Enabled {
    }
  }
  n366 = property on="On/Off" class="Bool (strict)"("Visible"=w14) -> ()  [unwired: 2 in, 2 out]
  n367 = property on="Motor" class="Clust (strict)"("Visible"=w14) -> ()  [unwired: 2 in, 2 out]
  n368 = property on="Progress" class="Clust (strict)"("Visible"=w14) -> ()  [unwired: 2 in, 2 out]
  n369 = property on="Test Ring" class="Ring (strict)"("Visible"=w14) -> ()  [unwired: 2 in, 2 out]
  n370 = property on="Rev/Fwd" class="Clust (strict)"("Visible"=w14) -> ()  [unwired: 2 in, 2 out]
  n371 = property on="Camera Settings" class="Clust (strict)"("Visible"=w14) -> ()  [unwired: 2 in, 2 out]
  n372 = local write "DB Camera Config"(w14) -> ()
  n373 = local write "Command Params"(string[][] [] ("Command Params")) -> ()
  n374 = global write "WPI_DashboardLogging Global.vi" "Recording"(w22) -> ()
  n375 = local write "Rec Mode"(w22) -> ()
  n376 = while {
    tunnel: u16 1741 ("timeout ms (25000)") -> [w625]
    stop <- FALSE stop-if-true
    n377 = TCP Create Listener(10:w625) -> (0:w624:errorcluster, 3:w626:refnum<k5>)  [unwired: 4 in, 1 out]
    n378 = case shown="No Error" w624 {
      selector: w624 -> [w628 _]
      tunnel: w626 -> [w629 _]
      frame No Error {
        n379 = while {
          tunnel: w629 -> [w632]
          tunnel: w628 -> [w631]
          stop <- FALSE stop-if-true
          n380 = TCP Wait On Listener(8:w631, 11:w632) -> (0:w633:errorcluster, 4:w634:refnum<k5>)  [unwired: 2 in, 3 out]
          n381 = local write "TCP"(w634) -> ()
          n382 = case shown="No Error" w633 {
            frame No Error {
            }
            frame Error {
              n383 = Wait (ms)(milliseconds to wait=u32 1000) -> ()  [unwired: 1 out]
            }
          }
        }
      }
      frame Error {
        n384 = Wait (ms)(milliseconds to wait=u32 1000) -> ()  [unwired: 1 out]
      }
    }
  }
  n385 = local write "Command Selection"(u16 0 ("milliseconds to wait")) -> ()
